vi "Get Sheet Name (Sheet Ref).vi"(8 "error in (no error)":errorcluster, 11 "Sheet Reference":refnum<k24>) -> (0 "error out":errorcluster, 3 "Sheet Reference out":refnum<k24>, 6 "Sheet Name (Sheet1)":string="Sheet1")   [LabVIEW 2014]
uses:
  C:/Users/LENOVO/Desktop/CodeSpace GUI/LVExcel/Resources/net40/NPOI.dll
  Resources/net40/NPOI.dll
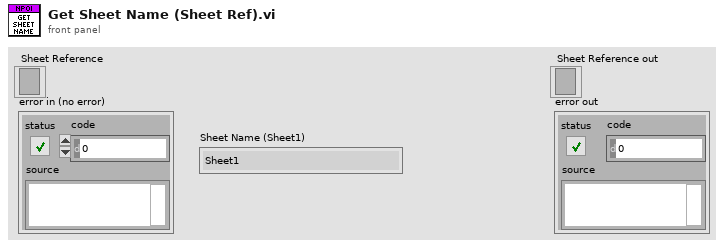
[diagram p1: front panel]
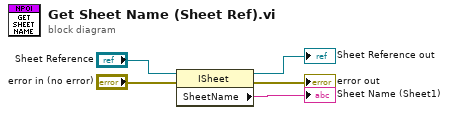
[diagram p0: block diagram]
diagram:
  n1 = property class="ISheet"(reference="Sheet Reference", error in="error in (no error)") -> (reference out=→"Sheet Reference out":refnum<k24>, error out=→"error out":errorcluster, "SheetName"=→"Sheet Name (Sheet1)":string)
